vi "Image Pixel Adjustment - SubVI.vi"(7 "Image Size":T1, 8 "error in":errorcluster, 9 "Set to Maximum":bool, 10 "Set to 512 x 300":bool, 11 "Set to AOI":bool) -> (0 "Pixels Out":i32[](array[numeric]), 1 "Error Out (no error)":errorcluster, 2 "Image Size 2":T1)   [LabVIEW 2014]
uses:
  Globals/Initilize Globals.vi
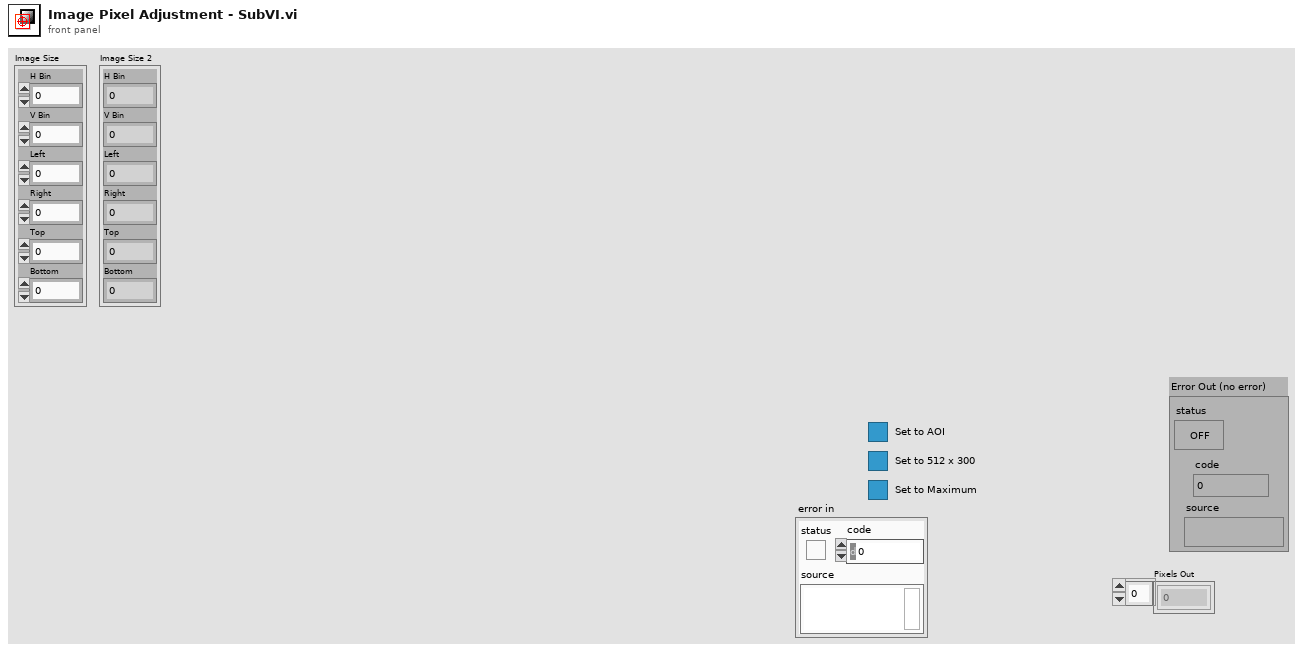
[diagram p1: front panel]
types:
  T1 = cluster{"H Bin":dbl, "V Bin":dbl, "Left":dbl, "Right":dbl, "Top":dbl, "Bottom":dbl}
  T2 = typedef "ROI Descriptor" = cluster{"Global Rectangle":i32[], "Contours":cluster{"ID":enum32{"External", "Internal"}, "Type":u32, "Coordinates":i32[]}[]}
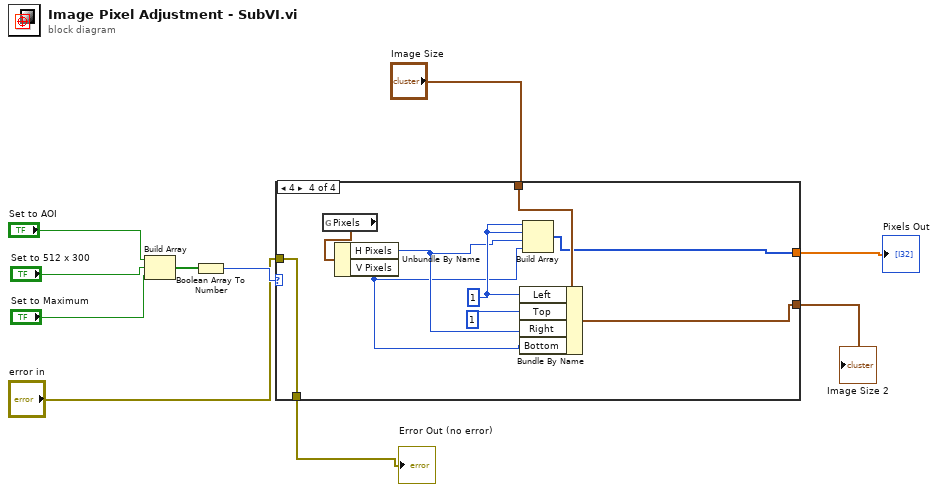
[diagram p0: block diagram]
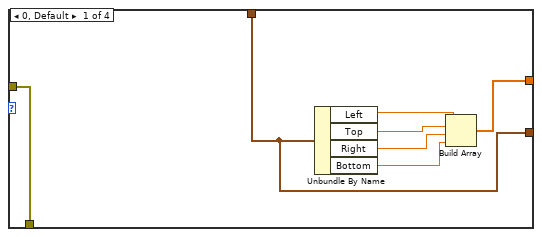
[diagram p2: hidden frame]
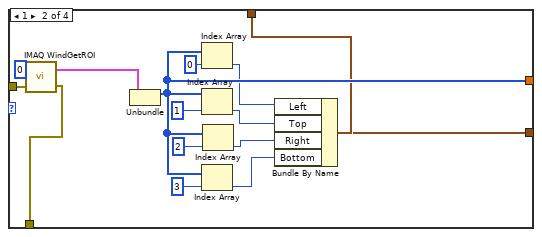
[diagram p3: hidden frame]
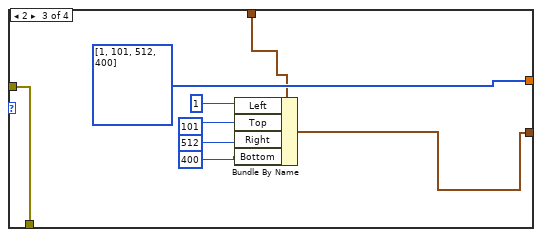
[diagram p4: hidden frame]
diagram:
  n1 = Build Array("Set to AOI", "Set to 512 x 300", "Set to Maximum") -> (w7:bool[])
  n2 = Boolean Array To Number(Boolean array=w7) -> (number=w6:u32)
  n3 = case shown="4" w6 {
    tunnel: "error in" -> [w17 w32 w40 w49]
    tunnel: [w12 w25 i32[] [1, 101, 512, 400] ("Global Rectangle") w42] -> w3
    tunnel: [w17 w30 w40 w49] -> w4
    tunnel: "Image Size" -> [w11 w19 w34 w47]
    tunnel: [w11 w18 w33 w41] -> w1
    frame 0, Default {
      n4 = Unbundle By Name(w11) -> ("Left"=w13:dbl, "Top"=w14:dbl, "Right"=w15:dbl, "Bottom"=w16:dbl)
      n5 = Build Array(w13, w14, w15, w16) -> (w12:dbl[])
    }
    frame 1 {
      n6 = call "IMAQ WindGetROI"("Window Number (0...15)"=0, "error in (no error)"=w32) -> ("ROI Descriptor"=w31:T2, "error out"=w30:errorcluster)  [unwired: 3 out]
      n7 = Unbundle(w31) -> ("Global Rectangle"=w25:i32[])  [unwired: 1 out]
      n8 = Index Array(array=w25, index=0) -> (element=w24:i32)
      n9 = Index Array(array=w25, index=1) -> (element=w23:i32)
      n10 = Index Array(array=w25, index=3) -> (element=w21:i32)
      n11 = Index Array(array=w25, index=2) -> (element=w22:i32)
      n12 = Bundle By Name(cluster=w19, "Left"=w24, "Top"=w23, "Right"=w22, "Bottom"=w21) -> (w18:T1)
    }
    frame 2 {
      n13 = Bundle By Name(cluster=w34, "Left"=1, "Top"=101, "Right"=512, "Bottom"=400) -> (w33:T1)
    }
    frame 4 {
      w45 = 1 ("Left")
      n14 = global read "Initilize Globals.vi" "Pixels"() -> (w46:cluster{"H Pixels":u32, "V Pixels":u32})
      n15 = Unbundle By Name(w46) -> ("H Pixels"=w44:u32, "V Pixels"=w43:u32)
      n16 = Bundle By Name(cluster=w47, "Left"=w45, "Top"=1, "Right"=w44, "Bottom"=w43) -> (w41:T1)
      n17 = Build Array(w45, w45, w44, w43) -> (w42:u32[])
    }
  }
  "Error Out (no error)" <- w4
  "Pixels Out" <- w3
  "Image Size 2" <- w1
